vi "Shfting.vi"() -> ()   [LabVIEW 2015]
panel:
  out "x << y":i32 format="%b"
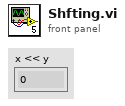
[diagram p1: front panel]
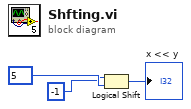
[diagram p0: block diagram]
diagram:
  n1 = Logical Shift(y=-1 ("x"), x=5) -> (x << y=→"x << y":i32)
